vi "Curtin1_LoadFile.vi"(11 "Files in":T1[](array[typedef])) -> (3 "Files out":T1[](array[typedef]))   [LabVIEW 2022 SP3]
uses:
  Curtin1_Label.ctl
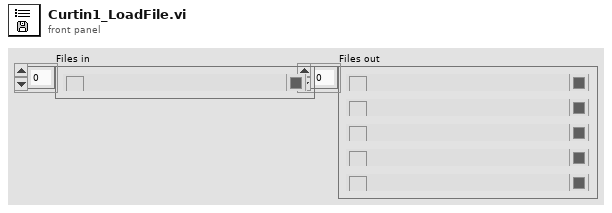
[diagram p1: front panel]
types:
  T1 = typedef "Curtin1_Label.ctl" = cluster{"Show?":bool, "Name":string, "Color":u32, "Path":path, "Show Notes":bool}
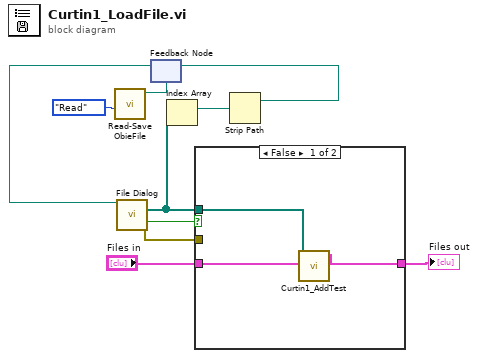
[diagram p0: block diagram]
diagram:
  n1 = call "Read-Save ObieFile.vi"("Task"=enum16{"Save", "Read"}."Read") -> ("DataPath Out"=w1:path)  [unwired: 8 in, 2 out]
  n2 = feedback #1(w1) -> (w2:path)
  n3 = call "File Dialog"("start path"=w2) -> ("selected paths"=w5:path[], "cancelled"=w8:bool, "error out"=w7:errorcluster)  [unwired: 11 in, 1 out]
  n4 = Index Array(array=w5) -> (element=w4:path)  [unwired: 1 in]
  n5 = case shown="False" w8 {
    tunnel: "Files in" -> [w13 w14]
    tunnel: [w12 w14] -> w10
    tunnel: w7 -> [_ _]
    tunnel: w5 -> [w11 _]
    frame False {
      n6 = call "Curtin1_AddTest.vi"("Old Files"=w13, "Selected Paths"=w11) -> ("New Files"=w12:T1[])  [unwired: 9 in]
    }
    frame True {
    }
  }
  "Files out" <- w10
  n7 = Strip Path(path=w4) -> (stripped path=w3:path)  [unwired: 1 out]
  n8 = feedback-in #1(w3) -> ()
